vi "CRYPIC Set BackImage.vi"(11 "pVIRef":refnum<vi>) -> ()   [LabVIEW 2013]
uses:
  CRYMainGlobal.vi
  Kernel32.DLL
panel:
  out "error out":errorcluster
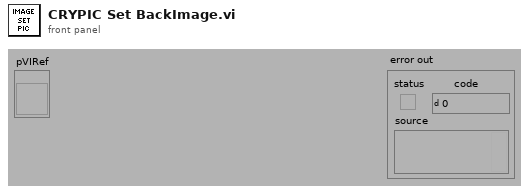
[diagram p1: front panel]
types:
  T1 = typedef "imagedata.ctl" = cluster{"image type":i32, "image depth":i32, "image":u8[], "mask":u8[], "colors":u32[], "Rectangle":cluster{"left":i16, "top":i16, "right":i16, "bottom":i16}}
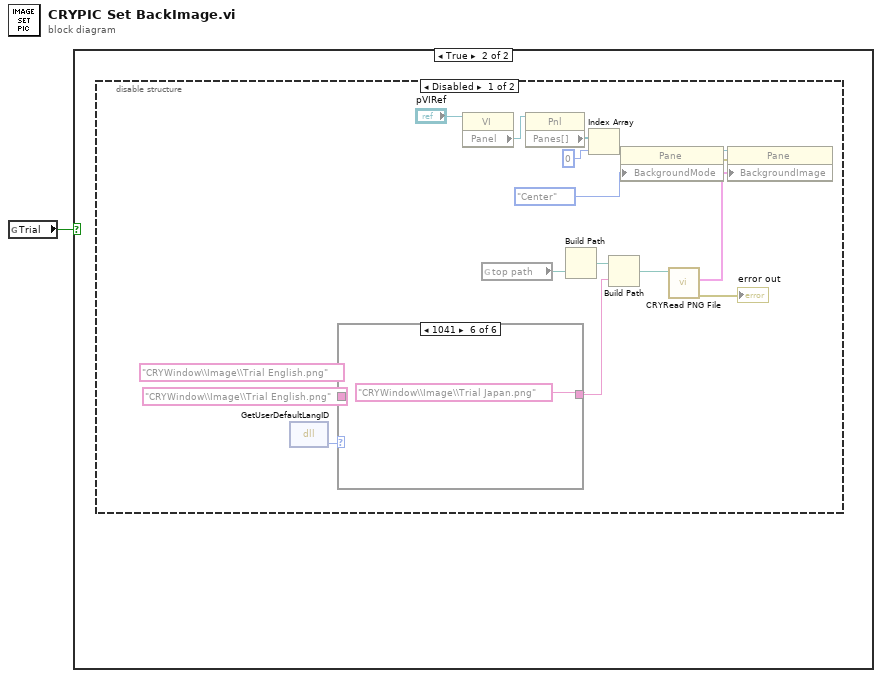
[diagram p0: block diagram]
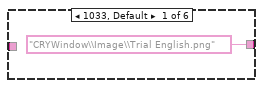
[diagram p3: hidden frame]
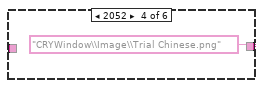
[diagram p6: hidden frame]
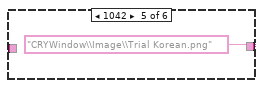
[diagram p7: hidden frame]
diagram:
  n1 = global read "CRYMainGlobal.vi" "Trial"() -> (w1:bool)
  n2 = case shown="True" w1 {
    frame False {
    }
    frame True {
      n3 = disable-structure shown="Disabled" {
        frame Disabled {
          (unwired) "CRYWindow\\Image\\Trial English.png"
          n4 = dll-call lib="kernel32.dll" fn="GetUserDefaultLangID"() -> ("return type"=w4:i32)  [unwired: 3 in, 2 out]
          n5 = case shown="1041" w4 {
            tunnel: ["CRYWindow\\Image\\Trial English.png" w19 w20 "CRYWindow\\Image\\Trial Chinese.png" "CRYWindow\\Image\\Trial Korean.png" "CRYWindow\\Image\\Trial Japan.png"] -> w3
            tunnel: "CRYWindow\\Image\\Trial English.png" -> [_ w19 w20 _ _ _]
            frame 1033, Default {
            }
            frame 1036 {
              # "1036"
            }
            frame 1031 {
              # "1031"
            }
            frame 2052 {
            }
            frame 1042 {
            }
            frame 1041 {
            }
          }
          n6 = property class="VI"(reference="pVIRef") -> ("Panel"=w17:refnum<vi>)  [unwired: 1 in, 2 out]
          n7 = global read "CRYMainGlobal.vi" "top path"() -> (w11:path)
          n8 = property class="Pnl"(reference=w17) -> ("Panes[]"=w16:refnum<vi>[])  [unwired: 1 in, 2 out]
          n9 = Build Path(name or relative path=w11) -> (appended path=w10:path)  [unwired: 1 out]
          n10 = Index Array(array=w16, index=0) -> (element=w14:refnum<vi>)
          n11 = Build Path(base path=w10, name or relative path=w3) -> (appended path=w7:path)
          n12 = property class="Pane"(reference=w14, "BackgroundMode"=enum16{"Stretch", "Center", "Tile"}."Center" ("Background Mode")) -> (reference out=w13:refnum<vi>, error out=w9:errorcluster)  [unwired: 1 in]
          n13 = call "CRYRead PNG File.vi"("path to PNG file"=w7) -> ("error out"=→"error out":errorcluster, "image data"=w6:T1)  [unwired: 8 in, 1 out]
          n14 = property class="Pane"(reference=w13, error in=w9, "BackgroundImage"=w6) -> ()  [unwired: 2 out]
        }
        frame Enabled {
        }
      }
    }
  }
